vi "ProgG_001_MG.vi"() -> ()   [LabVIEW 2021]
panel:
  out "2D array indicator 2":ext[][](array[numeric])=[[0.10000000000000000002, 1.0999999999999999999], [0.20000000000000000004, 1.20000000000000000004], [0.29999999999999999996, 1.29999999999999999996], [0.39999999999999999998, 1.4000000000000000001]]
  out "2D array indicator 1":i32[][](array[numeric])=[[12, 22], [13, 23], [14, 24], [15, 25]]
  in  "2D array control 2":ext[][](array[numeric])=[[1.1, 2.0999999999999999999], [1.20000000000000000004, 2.2], [1.29999999999999999996, 2.3], [1.4, 2.4000000000000000001]]
  in  "2D array control 1":i32[][](array[numeric])=[[11, 21], [12, 22], [13, 23], [14, 24]]
  out "1D array indicator 2":ext[](array[numeric])=[2.1100000000000000001, 3.22, 4.33]
  out "1D array indicator 1":i32[](array[numeric])=[0, 1, 2]
  in  "1D array control 2":ext[](array[numeric])=[1.11, 2.22, 3.33]
  in  "1D array control 1":i32[](array[numeric])=[1, 2, 3]
  out "Scalar indicator 2":ext=0.23000000000000000002
  in  "Scalar control 2":ext=1.23
  out "Scalar indicator 1":i32=2
  in  "Scalar control 1":i32=1
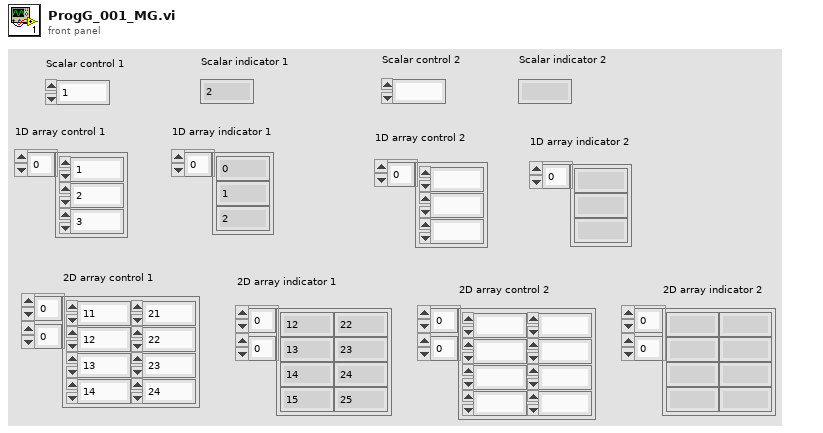
[diagram p1: front panel]
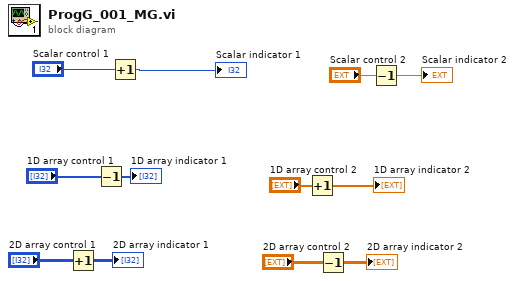
[diagram p0: block diagram]
diagram:
  n1 = Increment(x="2D array control 1") -> (x+1=→"2D array indicator 1":i32[][])
  n2 = Decrement(x="1D array control 1") -> (x-1=→"1D array indicator 1":i32[])
  n3 = Increment(x="Scalar control 1") -> (x+1=→"Scalar indicator 1":i32)
  n4 = Increment(x="1D array control 2") -> (x+1=→"1D array indicator 2":ext[])
  n5 = Decrement(x="2D array control 2") -> (x-1=→"2D array indicator 2":ext[][])
  n6 = Decrement(x="Scalar control 2") -> (x-1=→"Scalar indicator 2":ext)
